vi "mean_angle (SubVI).vi"(9 "quant":i32, 10 "angle 2":dbl, 11 "angle 1":dbl) -> (3 "angle out":dbl)   [LabVIEW 2015, in "PolyVIEW.lvclass"]
uses:
  PolyVIEW.lvclass
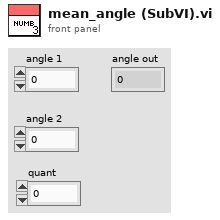
[diagram p1: front panel]
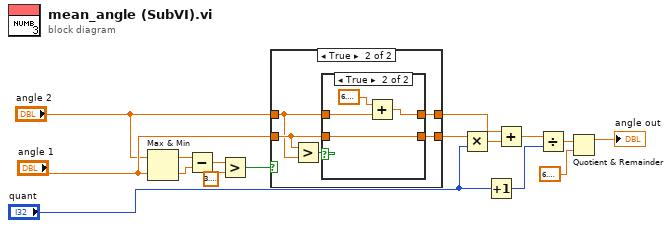
[diagram p0: block diagram]
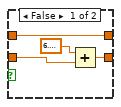
[diagram p3: hidden frame]
diagram:
  n1 = Max & Min(x="angle 2", y="angle 1") -> (max(x,y)=w3:dbl, min(x,y)=w4:dbl)
  n2 = Subtract(x=w3, y=w4) -> (x-y=w5:dbl)
  n3 = Greater?(x=w5, y=3.141592653589793) -> (0:w7:bool)
  n4 = case shown="True" w7 {
    tunnel: "angle 1" -> [w18 w22]
    tunnel: "angle 2" -> [w17 w21]
    tunnel: [w18 w20] -> w8
    tunnel: [w17 w19] -> w9
    frame False {
    }
    frame True {
      n5 = Greater?(x=w22, y=w21) -> (0:w23:bool)
      n6 = case shown="True" w23 {
        tunnel: w22 -> [w26 w31]
        tunnel: w21 -> [w24 w30]
        tunnel: [w25 w31] -> w20
        tunnel: [w24 w28] -> w19
        frame False {
          n7 = Add(x=6.283185307179586, y=w26) -> (x+y=w25:dbl)
        }
        frame True {
          n8 = Add(x=6.283185307179586, y=w30) -> (x+y=w28:dbl)
        }
      }
    }
  }
  n9 = Multiply(x=w8, y="quant") -> (x*y=w1:dbl)
  n10 = Increment(x="quant") -> (x+1=w10:i32)
  n11 = Add(x=w9, y=w1) -> (x+y=w2:dbl)
  n12 = Divide(x=w2, y=w10) -> (x/y=w11:dbl)
  n13 = Quotient & Remainder(x=w11, y=6.283185307179586) -> (x-y*floor(x/y)=→"angle out":dbl)  [unwired: 1 out]
